vi "복합연산.vi"() -> ()   [LabVIEW 2019]
panel:
  out "A6":dbl
  in  "A5":dbl
  in  "A4":dbl
  in  "A3":dbl
  in  "A2":dbl
  in  "A1":dbl
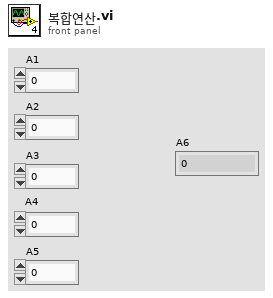
[diagram p1: front panel]
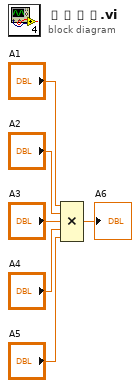
[diagram p0: block diagram]
diagram:
  n1 = Compound Arithmetic op=MULTIPLY("A1", "A2", "A3", "A4", "A5") -> (→"A6":dbl)
